vi "Read Data.vi"(5 "Wait Time(ms)":u32=50, 7 "Specified Num in":u8=1, 8 "error in (no error)":errorcluster caption="error in", 10 "Address":u16=4102 format="%.0x", 11 "Port Selection Info In":T1={"Port Name"="", "Amplifier Num"=1, "Baud Rate"=38400, "Char Formation"=enum."0"} {"Baud Rate" items=["38400"=38400, "19200"=19200, "9600"=9600, "115200"=0]; "Amplifier Num" max=31}) -> (0 "error out":errorcluster, 1 "Received Read Data":u8[](array[numeric]) format="%.0x", 2 "Data":u32[](array[numeric]), 3 "Port Selection Info Out":T1={"Port Name"="", "Amplifier Num"=1, "Baud Rate"=38400, "Char Formation"=enum."0"} {"Baud Rate" items=["38400"=38400, "19200"=19200, "9600"=9600, "115200"=0]; "Amplifier Num" max=31})   [LabVIEW 2014, in "ALPHA5 RS485.lvlib"]
uses:
  ALPHA5 RS485.lvlib
  typedefs/Port Selection Info.ctl
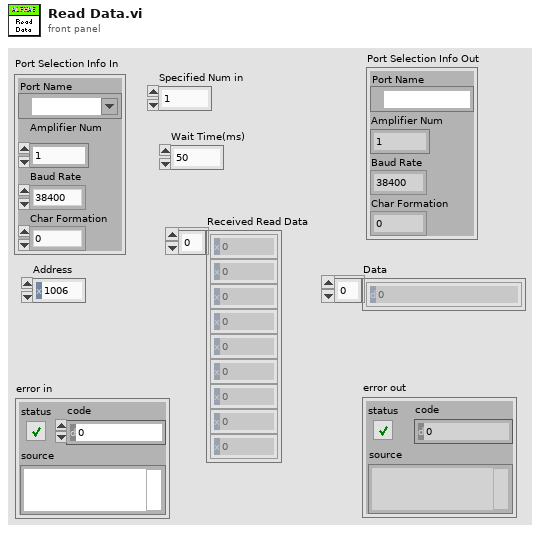
[diagram p1: front panel]
types:
  T1 = typedef "ALPHA5 RS485.lvlib/Port Selection Info.ctl" = cluster{"Port Name":refnum<visa-resource-name>, "Amplifier Num":u8, "Baud Rate":u32, "Char Formation":enum16{"0", "1", "2", "3", "4", "5"}}
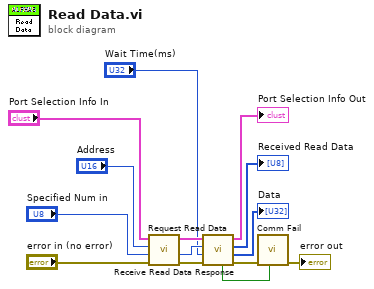
[diagram p0: block diagram]
diagram:
  n1 = call "Request Read Data.vi"("error in (no error)"="error in (no error)", "Specified Num in"="Specified Num in", "Address"="Address", "Port Selection Info"="Port Selection Info In") -> ("error out"=w9:errorcluster, "Specified Num out"=w11:u8, "Port Selection Info Out"=w12:T1)  [unwired: 5 in]
  n2 = call "Receive Read Data Response.vi"("error in (no error)"=w9, "Wait Time(ms)"="Wait Time(ms)", "Specified Num in"=w11, "Port Selection Info"=w12) -> ("error out"=w3:errorcluster, "Data"=→"Data":u32[], "Received Read Data"=→"Received Read Data":u8[], "Port Selection Info Out"=→"Port Selection Info Out":T1, "CRC Check?"=w1:bool)  [unwired: 2 in, 1 out]
  n3 = call "Comm Fail.vi"("CRC Match"=w1, "error in (no error)"=w3) -> ("error out"=→"error out":errorcluster)  [unwired: 9 in]
